vi "Find all uncalled vis.vi"() -> ()   [LabVIEW 2013]
panel:
  out "VIs in Project 2":string[](array[string])
  out "# of vis":i32
  out "Name":string
  out "VIs in Project":string[](array[string])
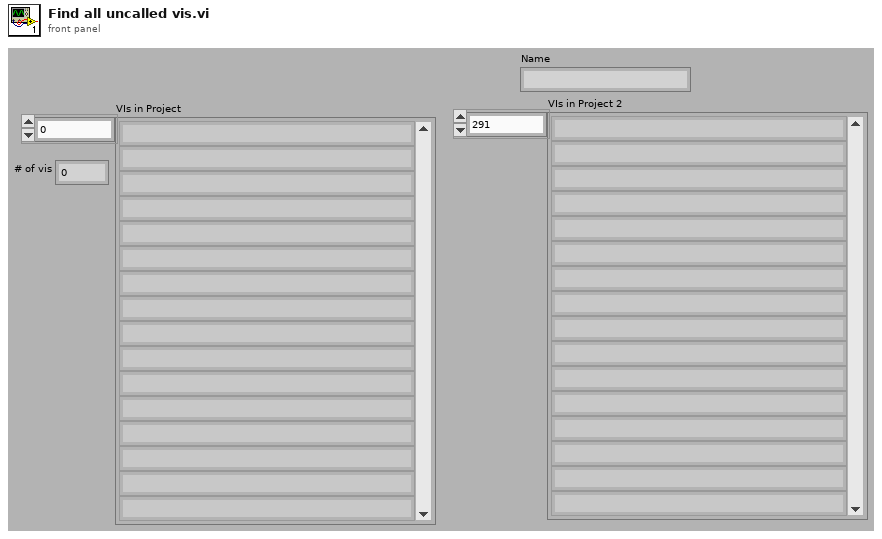
[diagram p1: front panel]
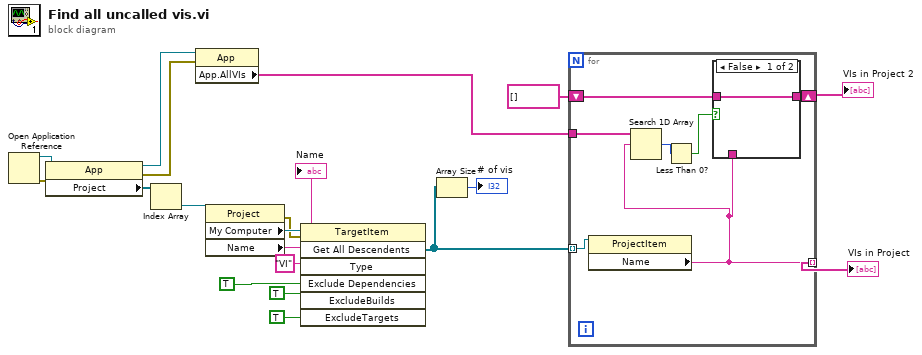
[diagram p0: block diagram]
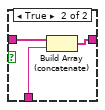
[diagram p2: hidden frame]
diagram:
  n1 = Open Application Reference() -> (0:w10:errorcluster, 3:w11:refnum<vi>)  [unwired: 1 in, 3 out]
  n2 = property class="App"(reference=w11, error in=w10) -> (reference out=w4:refnum<vi>, error out=w5:errorcluster, "Project"=w19:refnum<vi>[])
  n3 = Index Array(array=w19) -> (element=w18:refnum<vi>)  [unwired: 1 in]
  n4 = property class="App"(reference=w4, error in=w5) -> ("App.AllVIs"=w3:string[])  [unwired: 2 out]
  n5 = property class="Project"(reference=w18) -> (error out=w16:errorcluster, "My Computer"=w17:refnum<vi>, "Name"=→"Name":string)  [unwired: 1 in, 1 out]
  n6 = invoke class="TargetItem" method="Get All Descendents"(reference=w17, error in=w16, "Type"="VI", "Exclude Dependencies"=TRUE ("ExcludeDependencies"), "ExcludeBuilds"=TRUE, "ExcludeTargets"=TRUE ("ExcludeBuilds")) -> ("All Descendents"=w7:refnum<vi>[])  [unwired: 1 in, 6 out]
  n7 = Array Size(array=w7) -> (size(s)=→"# of vis":i32)
  n8 = for {
    tunnel: w7 -> [w26] mode=indexing
    tunnel: [w22] -> w12 mode=indexing
    tunnel: w3 -> [w25]
    shift-right: [w20] -> w1
    shift-left: string[] [] -> [w21]
    n9 = property class="ProjectItem"(reference=w26) -> ("Name"=w22:string)  [unwired: 1 in, 2 out]
    n10 = Search 1D Array(1D array=w25, element=w22) -> (index of element=w24:i32)  [unwired: 1 out]
    n11 = Less Than 0?(x=w24) -> (x < 0?=w23:bool)
    n12 = case shown="False" w23 {
      tunnel: w22 -> [_ w30]
      tunnel: w21 -> [w27 w29]
      tunnel: [w27 w28] -> w20
      frame False {
      }
      frame True {
        n13 = Build Array (concatenate)(w29, w30) -> (w28:string[])
      }
    }
  }
  "VIs in Project" <- w12
  "VIs in Project 2" <- w1
